vi "tm_getnextframe.vi"(6 "Image Type":u32, 7 "Timeout":i32=-1, 8 "error in (no error)":errorcluster, 9 "Image":T1, 10 "Buffer":u16[][](array[numeric]), 11 "Handle in":u32) -> (0 "error out":errorcluster, 2 "New Image":T1, 3 "Handle out":u32)   [LabVIEW 2012]
uses:
  tmcamcon.dll
  <vilib>/vision/Image Controls.llb/IMAQ Image.ctl
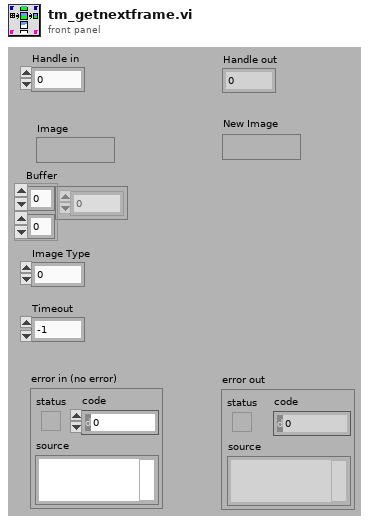
[diagram p1: front panel]
types:
  T1 = typedef "IMAQ Image.ctl" = refnum<image>
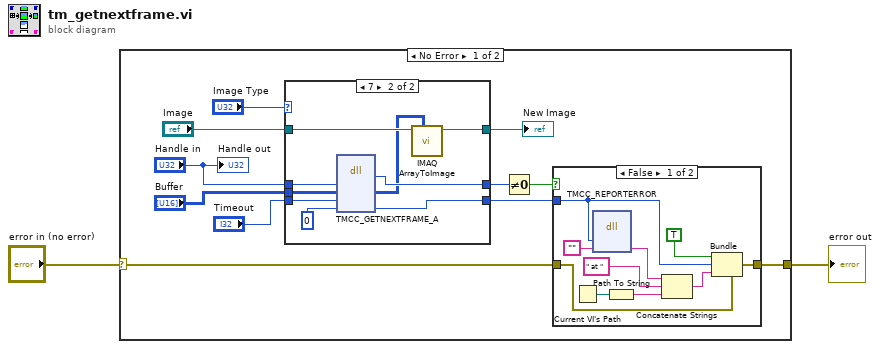
[diagram p0: block diagram]
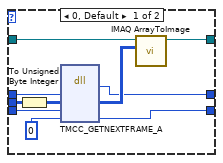
[diagram p3: hidden frame]
diagram:
  n1 = case shown="No Error" "error in (no error)" {
    selector: "error in (no error)" -> [w10 w44]
    tunnel: [w9 w44] -> w2
    frame No Error {
      n2 = case shown="7" "Image Type" {
        tunnel: [w34 w43] -> w13
        tunnel: "Image" -> [w33 w42]
        tunnel: "Handle in" -> [w32 w41]
        tunnel: "Buffer" -> [w31 w40]
        tunnel: [w28 w38] -> w5
        tunnel: [w27 w36] -> w4
        tunnel: "Timeout" -> [w25 w35]
        frame 0, Default {
          n3 = To Unsigned Byte Integer(number=w31) -> (unsigned 8bit integer=w30:u8[][])
          n4 = dll-call lib="tmcamcon.dll" fn="TMCC_GETNEXTFRAME_A"("index"=w32, "imgarray"=w30, "timeout"=w25, "Erval"=0) -> ("return type"=w28:u32, "imgarray"=w29:u8[][], "Erval"=w27:i32)  [unwired: 5 in, 2 out]
          n5 = call "IMAQ ArrayToImage"("Image Pixels (U8)"=w29, "Image"=w33) -> ("Image Out"=w34:T1)  [unwired: 8 in, 1 out]
        }
        frame 7 {
          n6 = dll-call lib="tmcamcon.dll" fn="TMCC_GETNEXTFRAME_A"("index"=w41, "imgarray"=w40, "timeout"=w35, "Erval"=0) -> ("return type"=w38:u32, "imgarray"=w37:u16[][], "Erval"=w36:i32)  [unwired: 5 in, 2 out]
          n7 = call "IMAQ ArrayToImage"("Image Pixels (U16)"=w37, "Image"=w42) -> ("Image Out"=w43:T1)  [unwired: 8 in, 1 out]
        }
      }
      "New Image" <- w13
      n8 = Not Equal To 0?(x=w5) -> (x != 0?=w11:bool)
      n9 = case shown="False" w11 {
        tunnel: w10 -> [w23 w24]
        tunnel: [w22 w24] -> w9
        tunnel: w4 -> [w16 _]
        frame False {
          n10 = Current VI's Path() -> (path=w21:path)
          n11 = dll-call lib="tmcamcon.dll" fn="TMCC_REPORTERROR"("error"=w16, "buf"="") -> ("buf"=w15:string)  [unwired: 5 in, 2 out]
          n12 = Path To String(path=w21) -> (string=w17:string)
          n13 = Concatenate Strings(w15, " at ", w17) -> (w20:string)
          n14 = Bundle(cluster=w23, "status"=TRUE, "code"=w16, "source"=w20) -> (w22:errorcluster)
        }
        frame True {
        }
      }
      "Handle out" <- "Handle in"
    }
    frame Error {
    }
  }
  "error out" <- w2
